vi "_01_Slide-1 Structure of FGV.vi"() -> ()   [LabVIEW 2020]
panel:
  out "String":string
  out "error out":errorcluster
  in  "error in (no error)":errorcluster
  in  "Enum":enum16{"Start", "Stop"}(ring)
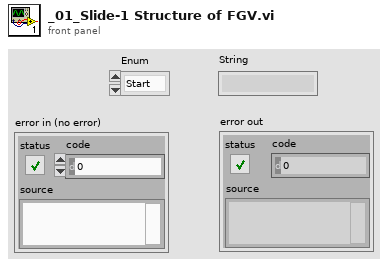
[diagram p1: front panel]
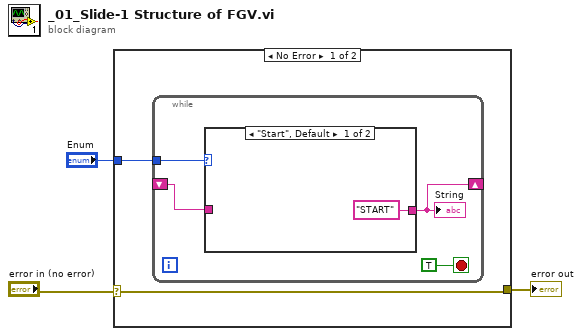
[diagram p0: block diagram]
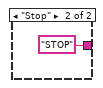
[diagram p2: hidden frame]
diagram:
  n1 = case shown="No Error" "error in (no error)" {
    selector: "error in (no error)" -> [w4 _]
    tunnel: "Enum" -> [w5 _]
    tunnel: [w4 _] -> w1
    frame No Error {
      n2 = while {
        tunnel: w5 -> [w9]
        shift-right: [w8] -> _
        shift-left: _ -> [w7]
        stop <- TRUE stop-if-true
        n3 = case shown="\"Start\", Default" w9 {
          tunnel: ["START" "STOP"] -> w8
          tunnel: w7 -> [_ _]
          frame "Start", Default {
          }
          frame "Stop" {
          }
        }
        "String" <- w8
      }
    }
    frame Error {
    }
  }
  "error out" <- w1
